vi "Get Position.vi"() -> (2 "Position":string)   [LabVIEW 2017]
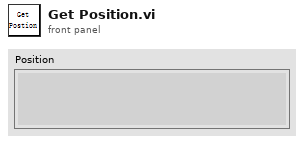
[diagram p1: front panel]
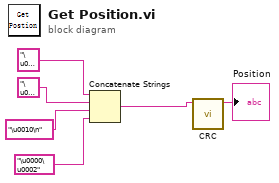
[diagram p0: block diagram]
diagram:
  n1 = Concatenate Strings("\u0001", "\u0003", "\u0010\n", "\u0000\u0002") -> (w1:string)
  n2 = call "CRC.vi"("字符串"=w1) -> ("连接的字符串"=→"Position":string)  [unwired: 9 in, 1 out]
